vi "Dequeue and Write to binary.vi"(0 "Queue name":string="Data", 1 "Queue data type":cluster{"Numeric":dbl, dbl, dbl, dbl, dbl}, 2 "Absolute file path of CSV":path=path "/home/lvuser", 3 "Error In":errorcluster, 4 "Record data":bool) -> (5 "error out":errorcluster)   [LabVIEW 2018]
panel:
  out "Queue empty":bool
  in  "Stop":bool
  out "Elements in queue":i32(slide) scale=0.0..10.0
  out "Elements stored":i32(slide) scale=0.0..10.0
  # "INPUTS"
  # "PURPOSE\nThis VI dequeues elements from queue 'Queue name', and writes them to a CSV file in location 'Absolute file path of CSV'..\n\nUSE\nOpen the block diagram and verify the data type of the queue matches that of the portion of the calling VI that enqueues the data being dequeued by this VI. If it does not then adjust portions (1) and (2) of the block diagram accordingly."
  # "OUTPUTS"
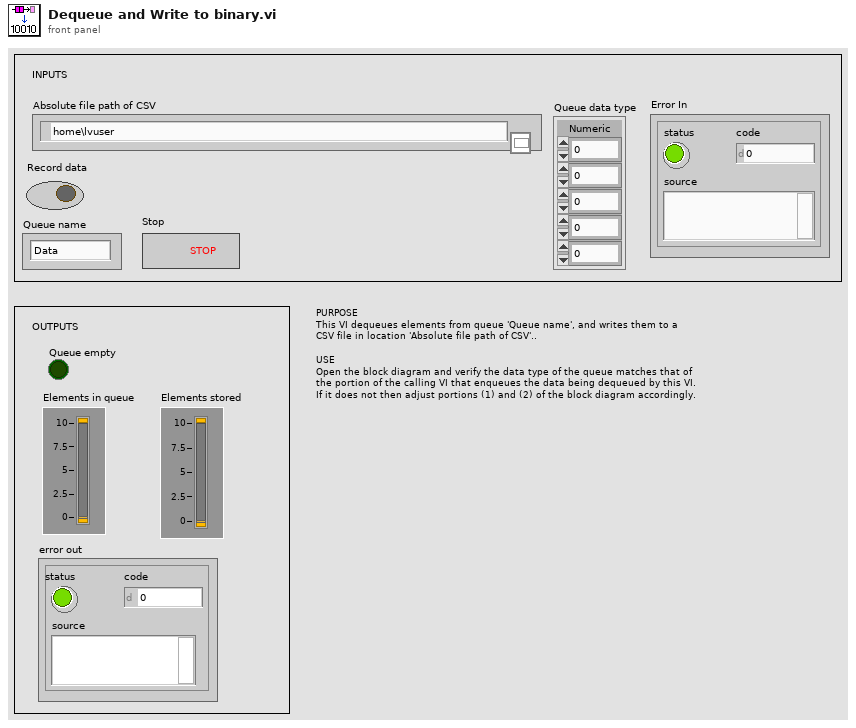
[diagram p1: front panel]
types:
  T1 = enum16{"big-endian, network order", "native, host order", "little-endian"}
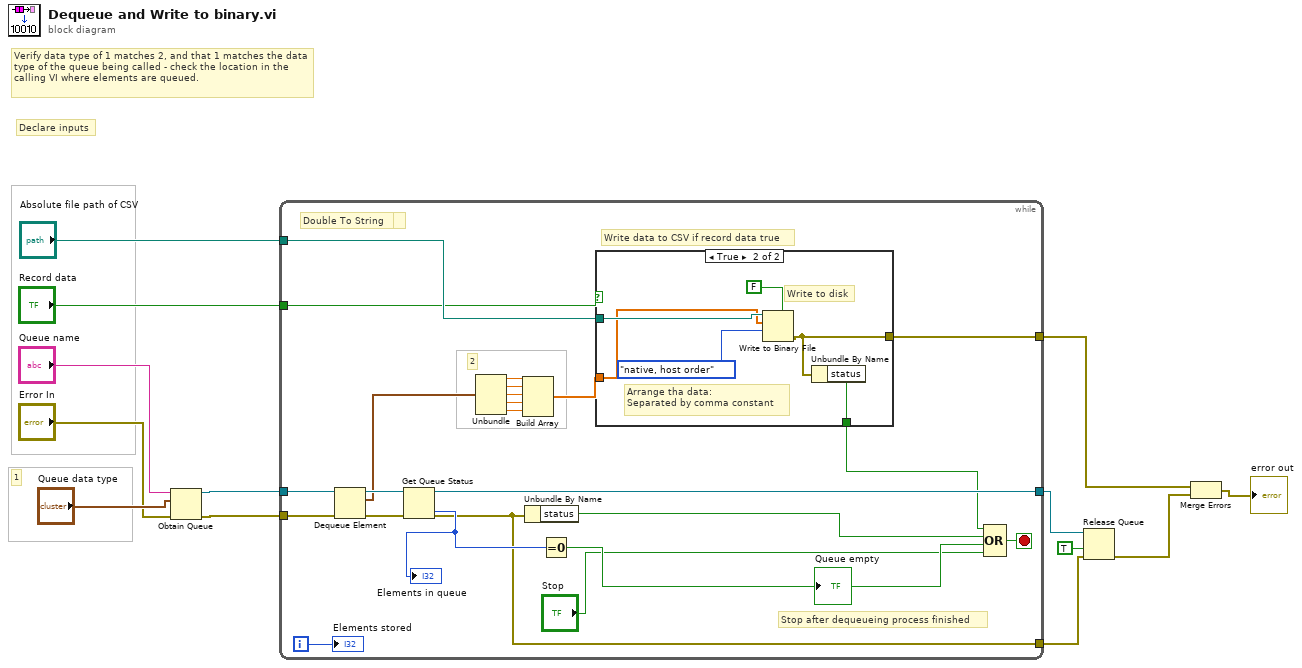
[diagram p0: block diagram]
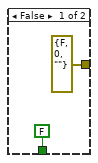
[diagram p2: hidden frame]
diagram:
  # "Declare inputs"
  # "1"
  # "Verify data type of 1 matches 2, and that 1 matches the data type of the queue being called - check the location in the calling VI where elements are queued."
  n1 = Obtain Queue(name (unnamed)="Queue name", element data type="Queue data type", error in (no error)="Error In") -> (queue out=w10:refnum<queue>, error out=w9:errorcluster)  [unwired: 2 in, 1 out]
  n2 = while {
    tunnel: w10 -> [w35]
    tunnel: [w31] -> w12
    tunnel: w9 -> [w28]
    tunnel: [w26] -> w7
    tunnel: "Absolute file path of CSV" -> [w23]
    tunnel: [w20] -> w2
    tunnel: "Record data" -> [w19]
    i -> [w29]
    stop <- w36 stop-if-true
    # "Write data to CSV if record data true"
    # "2"
    # "Data Logging Loop"
    # "Stop after dequeueing process finished"
    # "Double To String"
    n3 = Dequeue Element(queue=w35, error in (no error)=w28) -> (queue out=w33:refnum<queue>, element=w27:cluster{"Numeric":dbl, dbl, dbl, dbl, dbl}, error out=w32:errorcluster)  [unwired: 1 in, 1 out]
    n4 = Get Queue Status(queue=w33, error in (no error)=w32) -> (queue out=w31:refnum<queue>, error out=w26:errorcluster, # elements in queue=w30:i32)  [unwired: 1 in, 5 out]
    "Elements in queue" <- w30
    n5 = Unbundle(w27) -> ("Numeric"=w18:dbl, w17:dbl, w16:dbl, w15:dbl, w14:dbl)
    n6 = Build Array(w18, w17, w16, w15, w14) -> (w22:dbl[])
    n7 = Unbundle By Name(w26) -> ("status"=w34:bool)
    n8 = Equal To 0?(x=w30) -> (x = 0?=w25:bool)
    "Queue empty" <- w25
    n9 = case shown="True" w19 {
      tunnel: w23 -> [_ w43]
      tunnel: w22 -> [_ w42]
      tunnel: [errorcluster {"status"=FALSE, "code"=0, "source"=""} ("error out") w41] -> w20
      tunnel: [FALSE ("status") w44] -> w21
      frame False {
      }
      frame True {
        # "Write to disk"
        # "Arrange tha data:\nSeparated by comma constant"
        n10 = Write to Binary File(file (use dialog)=w43, data=w42, 5:FALSE ("prepend array or string size? (T)"), 9:T1."native, host order" ("byte order (0:big-endian, network order)")) -> (error out=w41:errorcluster)  [unwired: 2 in, 2 out]
        n11 = Unbundle By Name(w41) -> ("status"=w44:bool)
      }
    }
    n12 = Compound Arithmetic op=OR(w21, w34, w25, "Stop") -> (w36:bool)
    "Elements stored" <- w29
  }
  n13 = Release Queue(queue=w12, force destroy? (F)=TRUE, error in (no error)=w7) -> (error out=w4:errorcluster)  [unwired: 2 out]
  n14 = Merge Errors(w2, w4) -> (→"error out":errorcluster)
